vi "Start_WatchDog.vi"(8 "error in (no error)":errorcluster, 9 "Caller":refnum<queue>, 10 "ModToWatch":refnum<class "JQMHModule.lvclass">) -> (0 "error out":errorcluster)   [LabVIEW 2024, in "Watchdog.lvclass"]
uses:
  Watchdog.lvclass
  JQMHCore/Module/JQMHModule.lvclass
  C:/Github/JQMH/JQMHCore/Module/JQMHModule.lvclass
  Watchdog.lvclass/Watchdog.ctl
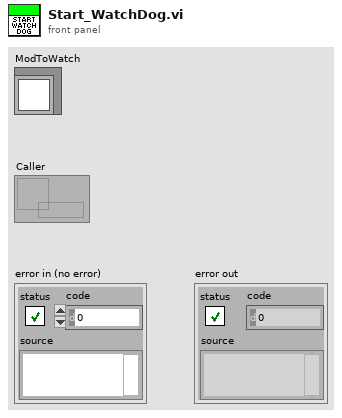
[diagram p1: front panel]
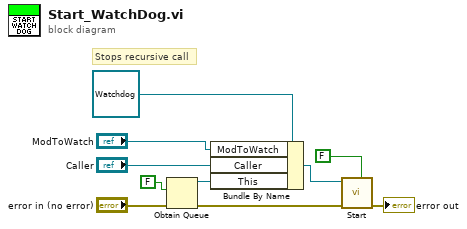
[diagram p0: block diagram]
diagram:
  # "Stops recursive call"
  n1 = Obtain Queue(element data type=FALSE, error in (no error)="error in (no error)") -> (queue out=w5:refnum<queue>, error out=w3:errorcluster)  [unwired: 3 in, 1 out]
  n2 = Bundle By Name(cluster=refnum<class "Watchdog.lvclass"> refnum ("Watchdog.lvclass"), "ModToWatch"="ModToWatch", "Caller"="Caller", "This"=w5) -> (w8:refnum<class "Watchdog.lvclass">)
  n3 = call "Start.vi"("Autoshutdown? (T)"=FALSE, "error in (no error)"=w3, "JQMHCore in"=w8) -> ("error out"=→"error out":errorcluster)  [unwired: 7 in, 1 out]
